vi "XYZStage-Stop all movement command.vi"(8 "Error In":errorcluster, 10 "Z Stage":T1, 11 "XYZ Stage config":T2={"COM port"="COM7", "Baudrate"=0, "Type"=""}) -> (0 "Error Out":errorcluster, 1 "Move XYZ command String":string)   [LabVIEW 2020]
uses:
  Typedefs/XY Stage config cluster.ctl
  Typedefs/Z Stage config cluster.ctl
  Typedefs/XYZ channel ring.ctl
  Typedefs/XYZ stage data.ctl
  Typedefs/XYZ stage states.ctl
  Global Variables/General Globals.vi
  Globals/gl_XYZStage globals.vi
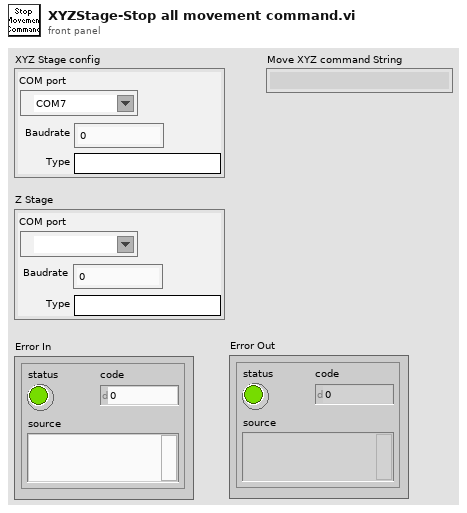
[diagram p1: front panel]
types:
  T1 = typedef "Z Stage config cluster.ctl" = cluster{"COM port":refnum<visa-resource-name>, "Baudrate":i32, "Type":string}
  T2 = typedef "XY Stage config cluster.ctl" = cluster{"COM port":refnum<visa-resource-name>, "Baudrate":i32, "Type":string}
  T3 = typedef "XYZ stage data.ctl" = cluster{"Command":T4, "Channel":T5, "X":sgl, "Y":sgl, "Z":sgl, "Speed":i32, "Zero":bool, "Use acknowledgement?":bool}
  T4 = typedef "XYZ stage states.ctl" = enum16{"Dequeue", "Initialize", "Read Position", "Read Speed Setting", "Move", "Set Max Speed", "Reset Axis", "Stop all movement"}
  T5 = typedef "XYZ channel ring.ctl" = string
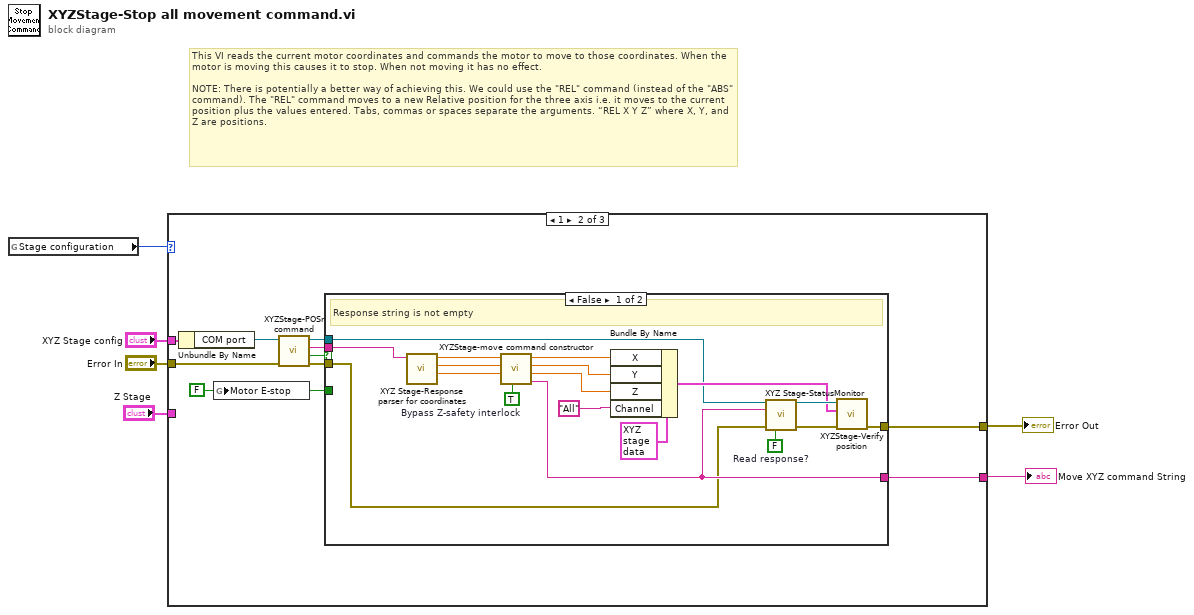
[diagram p0: block diagram]
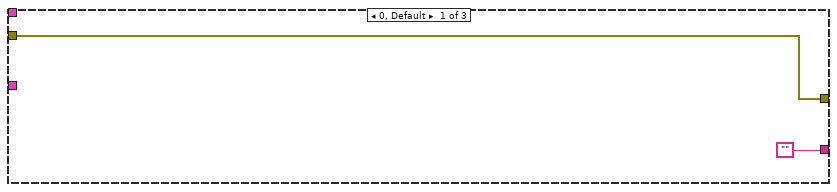
[diagram p2: hidden frame]
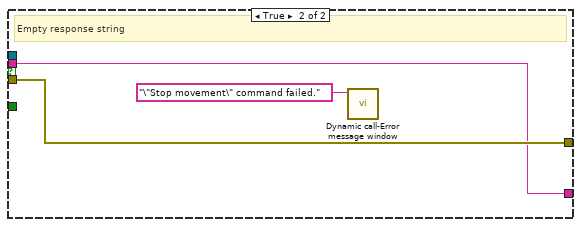
[diagram p3: hidden frame]
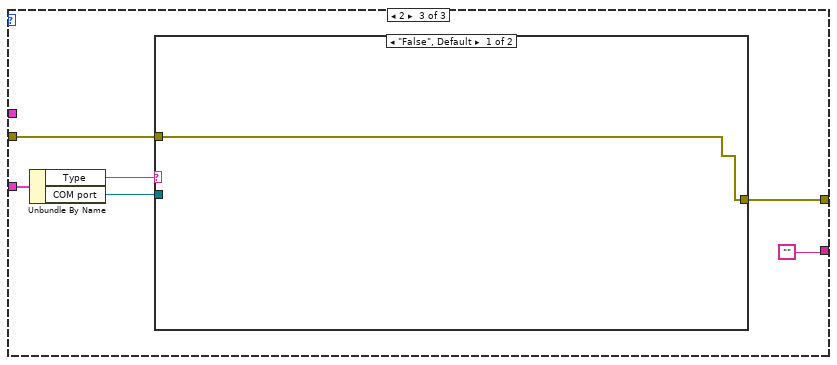
[diagram p4: hidden frame]
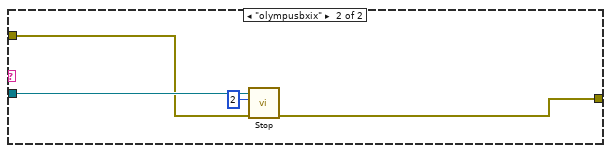
[diagram p5: hidden frame]
diagram:
  # "This VI reads the current motor coordinates and commands the motor to move to those coordinates. When the motor is moving this causes it to stop. When not moving it has no effect.\n\nNOTE: There is potentially a better way of achieving this. We could use the \"REL\" command (instead of the \"ABS\" command). The \"REL\" command moves to a new Relative position for the three axis i.e. it moves to the current position plus the values entered. Tabs, commas or spaces separate the arguments. “REL X Y Z” where X, Y, and Z are positions."
  n1 = global read "General Globals.vi" "Stage configuration"() -> (w2:i32)
  n2 = case shown="1" w2 {
    tunnel: "XYZ Stage config" -> [_ w18 _]
    tunnel: [w8 w17 w41] -> w5
    tunnel: ["" w16 ""] -> w4
    tunnel: "Error In" -> [w8 w14 w42]
    tunnel: "Z Stage" -> [_ _ w45]
    frame 0, Default {
    }
    frame 1 {
      w9 = FALSE ("Motor E-stop")
      n3 = Unbundle By Name(w18) -> ("COM port"=w15:refnum<visa-resource-name>)
      n4 = global write "gl_XYZStage globals.vi" "Motor E-stop"(w9) -> ()
      n5 = call "XYZStage-POSr command.vi"("Error in"=w14, "VISA Refnum in"=w15) -> ("Error out"=w13:errorcluster, "Empty response string"=w10:bool, "read string"=w11:string, "VISA Refnum out"=w12:refnum<visa-resource-name>)  [unwired: 6 in]
      n6 = case shown="False" w10 {
        tunnel: [w35 w39] -> w17
        tunnel: [w23 w38] -> w16
        tunnel: w13 -> [w21 w39]
        tunnel: w12 -> [w20 _]
        tunnel: w11 -> [w19 w38]
        tunnel: w9 -> [_ _]
        frame False {
          w22 = TRUE  # Bypass Z-safety interlock
          w33 = FALSE  # Read response?
          # "Response string is not empty"
          n7 = call "XYZ Stage-Response parser for coordinates.vi"("Filtered response string (no CR)"=w19) -> ("Z"=w27:sgl, "Y"=w28:sgl, "X"=w29:sgl)  [unwired: 7 in, 1 out]
          n8 = call "XYZStage-move command constructor.vi"("Bypass Z-safety interlock"=w22, "Z"=w27, "Y"=w28, "X"=w29) -> ("Move command"=w23:string, "Adjusted Z"=w24:sgl, "Adjusted Y"=w25:sgl, "Adjusted X"=w26:sgl)  [unwired: 3 in, 1 out]
          n9 = Bundle By Name(cluster=T3 {"Command"=enum."Stop all movement", "Channel"="", "X"=0.0, "Y"=0.0, "Z"=0.0, "Speed"=0, "Zero"=TRUE, "Use acknowledgement?"=FALSE} ("XYZ Stage data"), "X"=w26, "Y"=w25, "Z"=w24, "Channel"=T5 "All") -> (w31:T3)
          n10 = call "XYZ Stage-StatusMonitor.vi"("VISA resource name"=w20, "string to write"=w23, "Error In"=w21, "Read response? (T)"=w33) -> ("VISA resource name out"=w34:refnum<visa-resource-name>, "Error Out"=w36:errorcluster)  [unwired: 7 in, 3 out]
          n11 = call "XYZStage-Verify position.vi"("error in (no error)"=w36, "XYZ Stage data"=w31, "XYZ Stage Port"=w34) -> ("error out"=w35:errorcluster)  [unwired: 8 in]
        }
        frame True {
          # "Empty response string"
          n12 = call "Dynamic call-Error message window.vi"("Error Message"="\"Stop movement\" command failed.") -> ()  [unwired: 10 in, 1 out]
        }
      }
    }
    frame 2 {
      n13 = Unbundle By Name(w45) -> ("Type"=w44:string, "COM port"=w43:refnum<visa-resource-name>)
      n14 = case shown="\"False\", Default" w44 {
        tunnel: w43 -> [_ w50]
        tunnel: w42 -> [w46 w49]
        tunnel: [w46 w48] -> w41
        frame "False", Default {
        }
        frame "olympusbxix" {
          n15 = call "Stop.vi"("error in (no error)"=w49, "Device Number (1)"=2, "VISA Resource Name"=w50) -> ("error out"=w48:errorcluster)  [unwired: 6 in, 2 out]
        }
      }
    }
  }
  "Move XYZ command String" <- w4
  "Error Out" <- w5
